vi "SubVI_Example_MemoryAllocationSequence.vi"(0 ".NET (Reference)":refnum<k24>, 1 "Num Buffers":i32=2 min=1 max=5 step=1, 5 "Fehler (Eingang, kein Fehler)":errorcluster caption="Error In") -> (14 "Bits/Pixel 2":i32=8, 15 "Width":i32, 16 "Serial Number":string, 17 "Height":i32, 18 "Memory ID":i32, 19 "Fehler (Ausgang)":errorcluster caption="Error Out")   [LabVIEW 2010]
uses:
  C:/Program Files (x86)/National Instruments/LabVIEW 2016/instr.lib/IDS/ueye.NET/uEyeDotNet.dll
  Program Files (x86)/National Instruments/LabVIEW 2016/instr.lib/IDS/ueye.NET/uEyeDotNet.dll
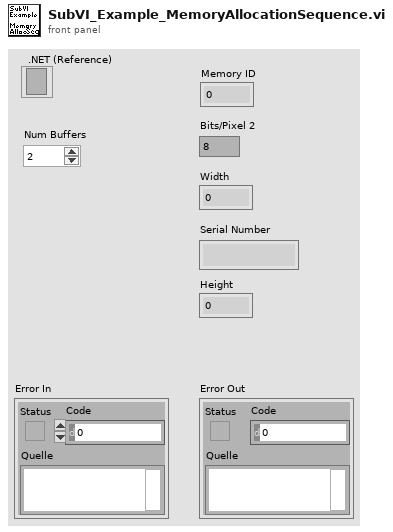
[diagram p1: front panel]
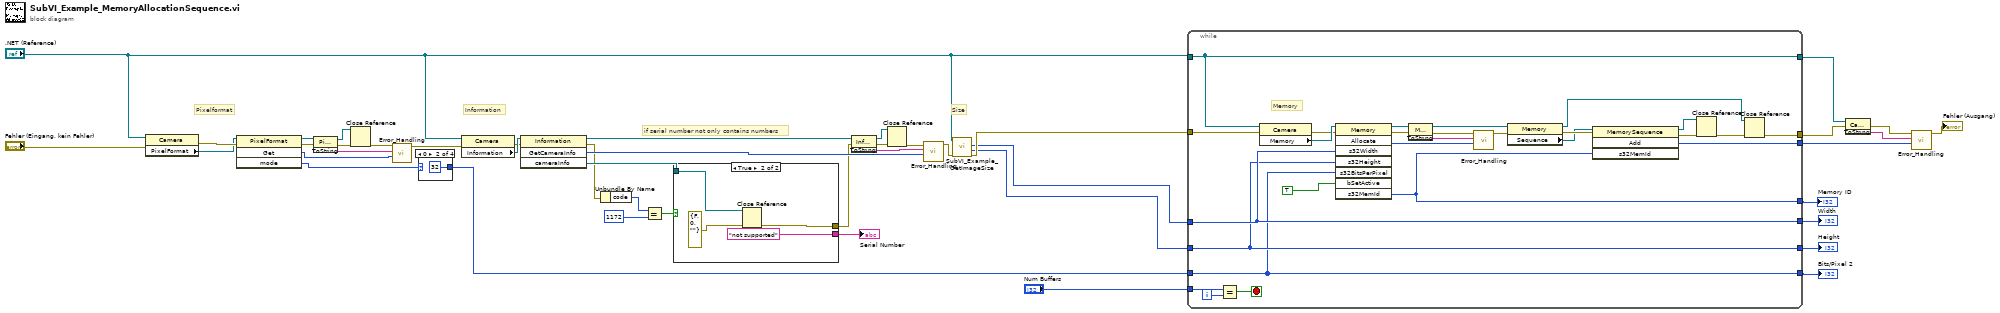
[diagram p0: block diagram]
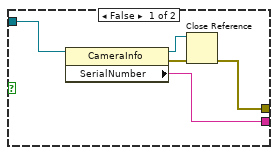
[diagram p2: hidden frame]
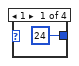
[diagram p3: hidden frame]
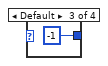
[diagram p4: hidden frame]
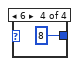
[diagram p5: hidden frame]
diagram:
  # "if serial number not only contains numbers"
  # "Information"
  # "Size"
  # "Pixelformat"
  n1 = property class="Camera"(reference=".NET (Reference)", error in="Fehler (Eingang, kein Fehler)") -> (error out=w32:errorcluster, "PixelFormat"=w31:refnum<k24>)  [unwired: 1 out]
  n2 = invoke class="PixelFormat" method="Get"(reference=w31, error in=w32) -> (reference out=w37:refnum<k24>, error out=w36:errorcluster, "Get"=w35:i32, "mode"=w28:i32)  [unwired: 2 in]
  n3 = invoke class="PixelFormat" method="ToString"(reference=w37, error in=w36) -> (reference out=w5:refnum<k24>, error out=w7:errorcluster, "ToString"=w34:string)  [unwired: 1 in]
  n4 = Close Reference(reference=w5, error in (no error)=w7) -> (error out=w6:errorcluster)
  n5 = call "Error_Handling.vi"("Error Code"=w35, "Error String"=w34, "Error In"=w6) -> ("Error Out"=w38:errorcluster)  [unwired: 8 in]
  n6 = case shown="0" w28 {
    tunnel: [24 32 -1 8] -> w20
    frame 1 {
    }
    frame 0 {
    }
    frame Default {
    }
    frame 6 {
    }
  }
  n7 = property class="Camera"(reference=".NET (Reference)", error in=w38) -> (error out=w29:errorcluster, "Information"=w30:refnum<k24>)  [unwired: 1 out]
  n8 = invoke class="Information" method="GetCameraInfo"(reference=w30, error in=w29) -> (reference out=w44:refnum<k24>, error out=w1:errorcluster, "GetCameraInfo"=w43:i32, "cameraInfo"=w24:refnum<k24>)  [unwired: 2 in]
  n9 = Unbundle By Name(w1) -> ("code"=w25:i32)
  n10 = Equal?(x=w25, y=1172) -> (x = y?=w27:bool)
  n11 = case shown="True" w27 {
    tunnel: [w50 w55] -> w22
    tunnel: w24 -> [w53 w54]
    tunnel: [w52 "not supported"] -> w23
    frame False {
      n12 = property class="CameraInfo"(reference=w53) -> (reference out=w49:refnum<k24>, error out=w51:errorcluster, "SerialNumber"=w52:string)  [unwired: 1 in]
      n13 = Close Reference(reference=w49, error in (no error)=w51) -> (error out=w50:errorcluster)
    }
    frame True {
      n14 = Close Reference(reference=w54, error in (no error)=errorcluster {"status"=FALSE, "code"=0, "source"=""} ("Error Out")) -> (error out=w55:errorcluster)
    }
  }
  "Serial Number" <- w23
  n15 = invoke class="Information" method="ToString"(reference=w44, error in=w22) -> (reference out=w2:refnum<k24>, error out=w4:errorcluster, "ToString"=w42:string)  [unwired: 1 in]
  n16 = Close Reference(reference=w2, error in (no error)=w4) -> (error out=w3:errorcluster)
  n17 = call "Error_Handling.vi"("Error Code"=w43, "Error String"=w42, "Error In"=w3) -> ("Error Out"=w12:errorcluster)  [unwired: 8 in]
  n18 = call "SubVI_Example_GetImageSize.vi"("Error In"=w12, ".NET (Reference)"=".NET (Reference)") -> ("Error Out"=w11:errorcluster, "Height"=w8:i32, "Width"=w9:i32)  [unwired: 6 in, 1 out]
  n19 = while {
    tunnel: "Num Buffers" -> [w82]
    tunnel: w11 -> [w70]
    tunnel: ".NET (Reference)" -> [w66]
    tunnel: w9 -> [w69]
    tunnel: w8 -> [w68]
    tunnel: w20 -> [w67]
    tunnel: [w69] -> w17
    tunnel: [w68] -> w18
    tunnel: [w67] -> w19
    tunnel: [w60] -> w15
    tunnel: [w66] -> w14
    tunnel: [w65] -> w16
    tunnel: [w64] -> w13
    i -> [w84]
    stop <- w83 stop-if-true
    # "Memory"
    n20 = Equal?(x=w82, y=w84) -> (x = y?=w83:bool)
    n21 = property class="Camera"(reference=w66, error in=w70) -> (error out=w80:errorcluster, "Memory"=w81:refnum<k24>)  [unwired: 1 out]
    n22 = invoke class="Memory" method="Allocate"(reference=w81, error in=w80, "s32Width"=w69, "s32Height"=w68, "s32BitsPerPixel"=w67, "bSetActive"=TRUE) -> (reference out=w73:refnum<k24>, error out=w72:errorcluster, "Allocate"=w74:i32, "s32MemId"=w65:i32)  [unwired: 2 in, 4 out]
    n23 = invoke class="Memory" method="ToString"(reference=w73, error in=w72) -> (reference out=w63:refnum<k24>, error out=w75:errorcluster, "ToString"=w76:string)  [unwired: 1 in]
    n24 = call "Error_Handling.vi"("Error Code"=w74, "Error String"=w76, "Error In"=w75) -> ("Error Out"=w71:errorcluster)  [unwired: 8 in]
    n25 = property class="Memory"(reference=w63, error in=w71) -> (reference out=w58:refnum<k24>, error out=w78:errorcluster, "Sequence"=w77:refnum<k24>)
    n26 = invoke class="MemorySequence" method="Add"(reference=w77, error in=w78, "s32MemId"=w65) -> (reference out=w59:refnum<k24>, error out=w62:errorcluster, "Add"=w64:i32)  [unwired: 1 in, 1 out]
    n27 = Close Reference(reference=w59, error in (no error)=w62) -> (error out=w61:errorcluster)
    n28 = Close Reference(reference=w58, error in (no error)=w61) -> (error out=w60:errorcluster)
  }
  "Bits/Pixel 2" <- w19
  "Height" <- w18
  "Width" <- w17
  "Memory ID" <- w16
  n29 = invoke class="Camera" method="ToString"(reference=w14, error in=w15) -> (error out=w39:errorcluster, "ToString"=w40:string)  [unwired: 1 in, 1 out]
  n30 = call "Error_Handling.vi"("Error Code"=w13, "Error String"=w40, "Error In"=w39) -> ("Error Out"=→"Fehler (Ausgang)":errorcluster)  [unwired: 8 in]
